vi "New Verify as Parameterized.vi"   [LabVIEW 2020, in "Caraya.Extension.lvlib"]
uses:
  Caraya.Extension.lvlib
  <vilib>/addons/_JKI Toolkits/Caraya/classes/Test/Test.lvclass
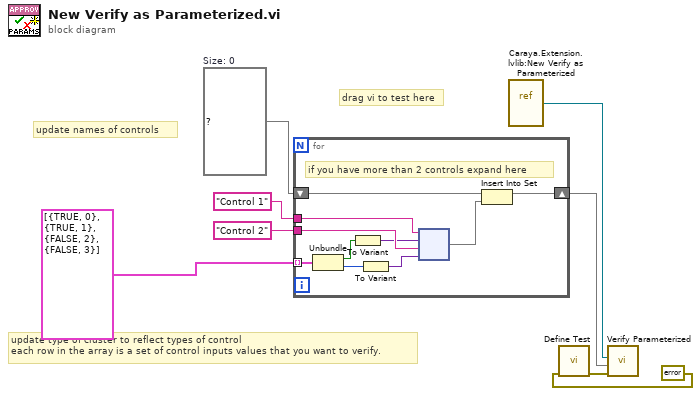
[diagram p0: block diagram]
diagram:
  w2 = set{map{string, variant}} {}  # Size: 0
  # "update type of cluster to reflect types of control\neach row in the array is a set of control inputs values that you want to verify."
  # "update names of controls"
  # "drag vi to test here"
  n1 = for {
    tunnel: "Control 1" -> [w18]
    tunnel: cluster{bool, i32}[] [{TRUE, 0}, {TRUE, 1}, {FALSE, 2}, {FALSE, 3}] -> [w16] mode=indexing
    tunnel: "Control 2" -> [w17]
    shift-right: [w10] -> w1
    shift-left: w2 -> [w9]
    # "if you have more than 2 controls expand here"
    n2 = Unbundle(w16) -> (w15:bool, w14:i32)
    n3 = To Variant(anything=w15) -> (Variant=w12:variant)
    n4 = To Variant(anything=w14) -> (Variant=w11:variant)
    n5 = node(w18, w12, w17, w11) -> (w13:map{string, variant})
    n6 = Insert Into Set(10:w13, 11:w9) -> (3:w10:set{map{string, variant}})  [unwired: 1 out]
  }
  n7 = vi-ref "Caraya.Extension.lvlib:New Verify as Parameterized.vi"() -> (w6:refnum<vi>)
  n8 = call <vilib>:"Define Test.vi"("error in (no error)"=errorcluster {"status"=FALSE, "code"=0, "source"=""}) -> ("error out"=w7:errorcluster)  [unwired: 9 in, 1 out]
  n9 = call "Verify Parameterized.vi"("error in"=w7, "ctl label -> value var"=w1, "VI Refnum"=w6) -> ()  [unwired: 7 in, 2 out]
